vi "SetJSONData.vi"(0 "reference in":refnum<class "BooleanControl.lvclass">, 1 "VI Reference":refnum<vi>, 2 "Value":string, 5 "error in (no error)":errorcluster) -> (14 "reference out":refnum<class "BooleanControl.lvclass">, 19 "error out":errorcluster)   [LabVIEW 2014, in "BooleanControl.lvclass"]
uses:
  BooleanControl.lvclass
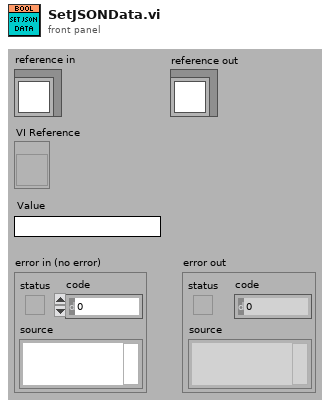
[diagram p1: front panel]
types:
  T1 = typedef "BooleanControl.lvclass/Attributes.ctl" = cluster{"Boolean ref":refnum<vi>, "Switching":bool, "Boolean Strings":string[], "Text":refnum<class "Text.lvclass">}
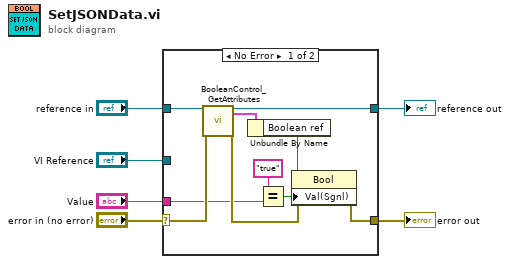
[diagram p0: block diagram]
diagram:
  n1 = case shown="No Error" "error in (no error)" {
    selector: "error in (no error)" -> [w16 w18]
    tunnel: [w15 w18] -> w5
    tunnel: [w11 w17] -> w3
    tunnel: "reference in" -> [w12 w17]
    tunnel: "Value" -> [w10 _]
    tunnel: "VI Reference" -> [_ _]
    frame No Error {
      n2 = call "BooleanControl_GetAttributes.vi"("reference in"=w12, "error in (no error)"=w16) -> ("reference out"=w11:refnum<class "BooleanControl.lvclass">, "Data"=w13:T1, "error out"=w14:errorcluster)  [unwired: 14 in, 1 out]
      n3 = Unbundle By Name(w13) -> ("Boolean ref"=w7:refnum<vi>)
      n4 = Equal?(x="true" ("y"), y=w10) -> (x = y?=w8:bool)
      n5 = property class="Bool"(reference=w7, error in=w14, "Val(Sgnl)"=w8) -> (error out=w15:errorcluster)  [unwired: 1 out]
    }
    frame Error {
    }
  }
  "error out" <- w5
  "reference out" <- w3
